vi "FTW-CodeGen-XNodeReply.vi"(0 "XNode Reply Type":T1) -> (4 "Reply":string[](array[string]))   [LabVIEW 2015]
uses:
  FTW-CodeGen-XNodeReplyType.ctl
panel:
  # "Inputs"
  # "Outputs"
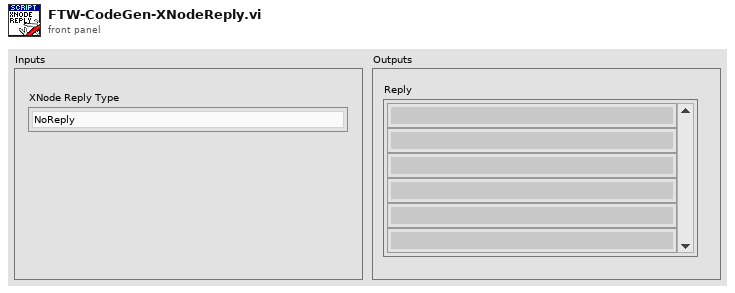
[diagram p1: front panel]
types:
  T1 = typedef "FTW-CodeGen-XNodeReplyType.ctl" = enum16{"NoReply", "ForceAdaptToInputs", "UpdateTerms", "GenCode", "GenCode+CosmeticUpdate"}
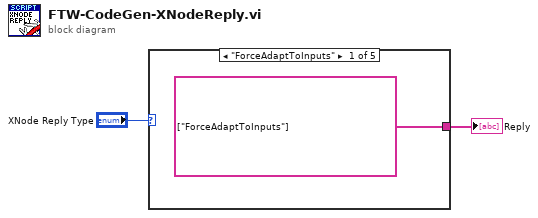
[diagram p0: block diagram]
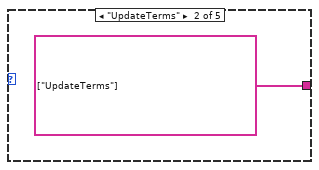
[diagram p2: hidden frame]
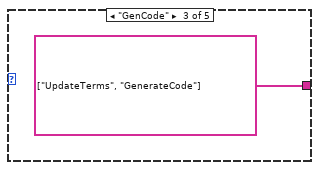
[diagram p3: hidden frame]
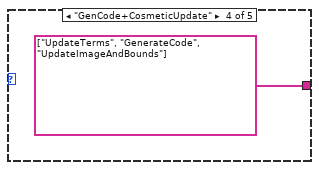
[diagram p4: hidden frame]
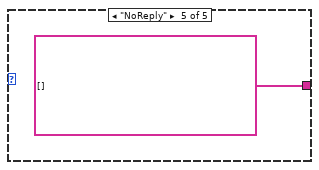
[diagram p5: hidden frame]
diagram:
  n1 = case shown="\"ForceAdaptToInputs\"" "XNode Reply Type" {
    tunnel: [string[] ["ForceAdaptToInputs"] ("Reply") string[] ["UpdateTerms"] ("Reply") string[] ["UpdateTerms", "GenerateCode"] ("Reply") string[] ["UpdateTerms", "GenerateCode", "UpdateImageAndBounds"] ("Reply") string[] [] ("Reply")] -> w1
    frame "ForceAdaptToInputs" {
    }
    frame "UpdateTerms" {
    }
    frame "GenCode" {
    }
    frame "GenCode+CosmeticUpdate" {
    }
    frame "NoReply" {
    }
  }
  "Reply" <- w1
